vi "DBCHandle.vi"() -> ()   [LabVIEW 2020]
panel:
  out "DBCHandle":u32 format="%x"
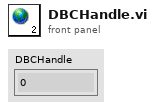
[diagram p1: front panel]
diagram:
